vi "Data_Collection.vi"() -> ()   [LabVIEW 2016]
uses:
  <vilib>/Analysis/3filter.llb/Filter Passband Type.ctl
  <vilib>/myRIO/Instrument Drivers/Onboard Devices/Accelerometer/typedefs/Accelerometer Reference.ctl
  <vilib>/myRIO/Common/Instrument Driver Framework/Utilities/typedefs/myRIO Generic Hardware Reference.ctl
  <vilib>/myRIO/Common/Instrument Driver Framework/Utilities/typedefs/Hardware Version Enum.ctl
  <vilib>/myRIO/Common/Instrument Driver Framework/Utilities/typedefs/myRIO v1.0 Reference.ctl
  <vilib>/myRIO/Common/Instrument Driver Framework/Utilities/typedefs/Generic FPGA Reference.ctl
  <vilib>/myRIO/Common/Instrument Driver Framework/myRIO v1.0/Accelerometer/typedefs/Accelerometer Channels List.ctl
  <vilib>/myRIO/Common/Instrument Driver Framework/myRIO v1.0/Accelerometer/typedefs/Accelerometer Channels Enum.ctl
  <vilib>/userdefined/High Color/nirio_resource_hc.ctl
  <vilib>/myRIO/Common/Instrument Driver Framework/Utilities/vis/Is FPGA Ref Available.vi
  <vilib>/myRIO/Common/Instrument Driver Framework/myRIO v1.0/Accelerometer/vis/myRIO v1.1 Open Accelerometer.vi
  <vilib>/myRIO/Instrument Drivers/Onboard Devices/Accelerometer/vis/Read.vi
  <vilib>/myRIO/Common/Instrument Driver Framework/Utilities/vis/Validate Channels.vi
  <vilib>/myRIO/Common/Instrument Driver Framework/myRIO v1.0/Accelerometer/vis/myRIO v1.0 Reserve Accelerometer.vi
  <vilib>/myRIO/Common/Instrument Driver Framework/myRIO v1.0/UART/vis/myRIO v1.0 Close UART.vi
  <vilib>/myRIO/Common/Instrument Driver Framework/myRIO v1.0/Resource Manager/vis/myRIO v1.0 Reserve Channel List.vi
  <vilib>/myRIO/Common/Instrument Driver Framework/myRIO v1.0/Accelerometer/vis/myRIO v1.0 Build MUX Configuration Accelerometer.vi
  <vilib>/myRIO/Common/Instrument Driver Framework/myRIO v1.0/Resource Manager/vis/myRIO v1.0 Reserve Channel.vi
  <vilib>/myRIO/Common/Instrument Driver Framework/myRIO v1.0/Resource Manager/vis/myRIO v1.0 Unreserve Channel.vi
  <vilib>/myRIO/Common/Instrument Driver Framework/myRIO v1.0/Resource Manager/vis/myRIO v1.0 Build Mutex Name.vi
  <vilib>/Utility/VariantDataType/GetNumericInfo.vi
  <vilib>/Utility/error.llb/Error Cluster From Error Code.vi
  <vilib>/myRIO/Common/Instrument Driver Framework/myRIO v1.0/myRIO v1.1 Open.vi
  <vilib>/myRIO/Common/Instrument Driver Framework/myRIO v1.0/Accelerometer/vis/myRIO v1.0 Get Scaling Constant Accelerometer.vi
  <vilib>/myRIO/Common/Instrument Driver Framework/Utilities/vis/IO Manager.vi
  <vilib>/myRIO/Common/Instrument Driver Framework/Utilities/vis/Configuration Manager.vi
  <vilib>/myRIO/Common/Instrument Driver Framework/myRIO v1.0/myRIO v1.0 Close.vi
  <vilib>/myRIO/Common/Instrument Driver Framework/myRIO v1.0/Accelerometer/vis/myRIO v1.0 Read Accelerometer.vi
  <vilib>/myRIO/Common/Instrument Driver Framework/Utilities/vis/FPGA Ref Manager.vi
  <vilib>/myRIO/Common/Instrument Driver Framework/myRIO v1.0/myRIO v1.0 Reset FPGA.vi
  <vilib>/myRIO/Common/Instrument Driver Framework/myRIO v1.0/IRQ/vis/myRIO v1.0 IRQ Info FGV.vi
  <vilib>/myRIO/Common/Instrument Driver Framework/myRIO v1.0/IRQ/vis/myRIO v1.0 Timer IRQ Info FGV.vi
  <vilib>/myRIO/Common/Instrument Driver Framework/myRIO v1.0/IRQ/vis/myRIO v1.0 ISR Agent.vi
  <vilib>/myRIO/Express VI/Onboard Devices/Accelerometer/Accelerometer Express VI.xnode
  <vilib>/myRIO/Instrument Drivers/Onboard Devices/Accelerometer/vis/myRIO Accelerometer Open.xnode
  <vilib>/Analysis/NI_AALBase.lvlib
  <vilib>/myRIO/Instrument Drivers/Onboard Devices/Accelerometer/Accelerometer.lvlib
  <vilib>/ptbypt/NI_PtbyPt.lvlib
  <vilib>/myRIO/Instrument Drivers/Utilities/Utilities.lvlib
panel:
  out "Collected output":dbl[](array[numeric])
  in  "N Samples":dbl
  out "Collected Data":dbl[][](array[numeric])
  in  "Stop Main":bool
  in  "Input Number":dbl
  out "Data as 1D":dbl[](array[numeric])
  out "Data as 2D":dbl[][](array[numeric])
  in  "Start Data Collect":bool
  out "error out":errorcluster
  out "Raw Values":T1(graph) caption="Waveform Chart"
  in  "Stop Data Collect":bool
  out "Pitch and Roll":cluster{"r":dbl, "p":dbl}(graph) caption="Waveform Chart"
  out "?":dbl
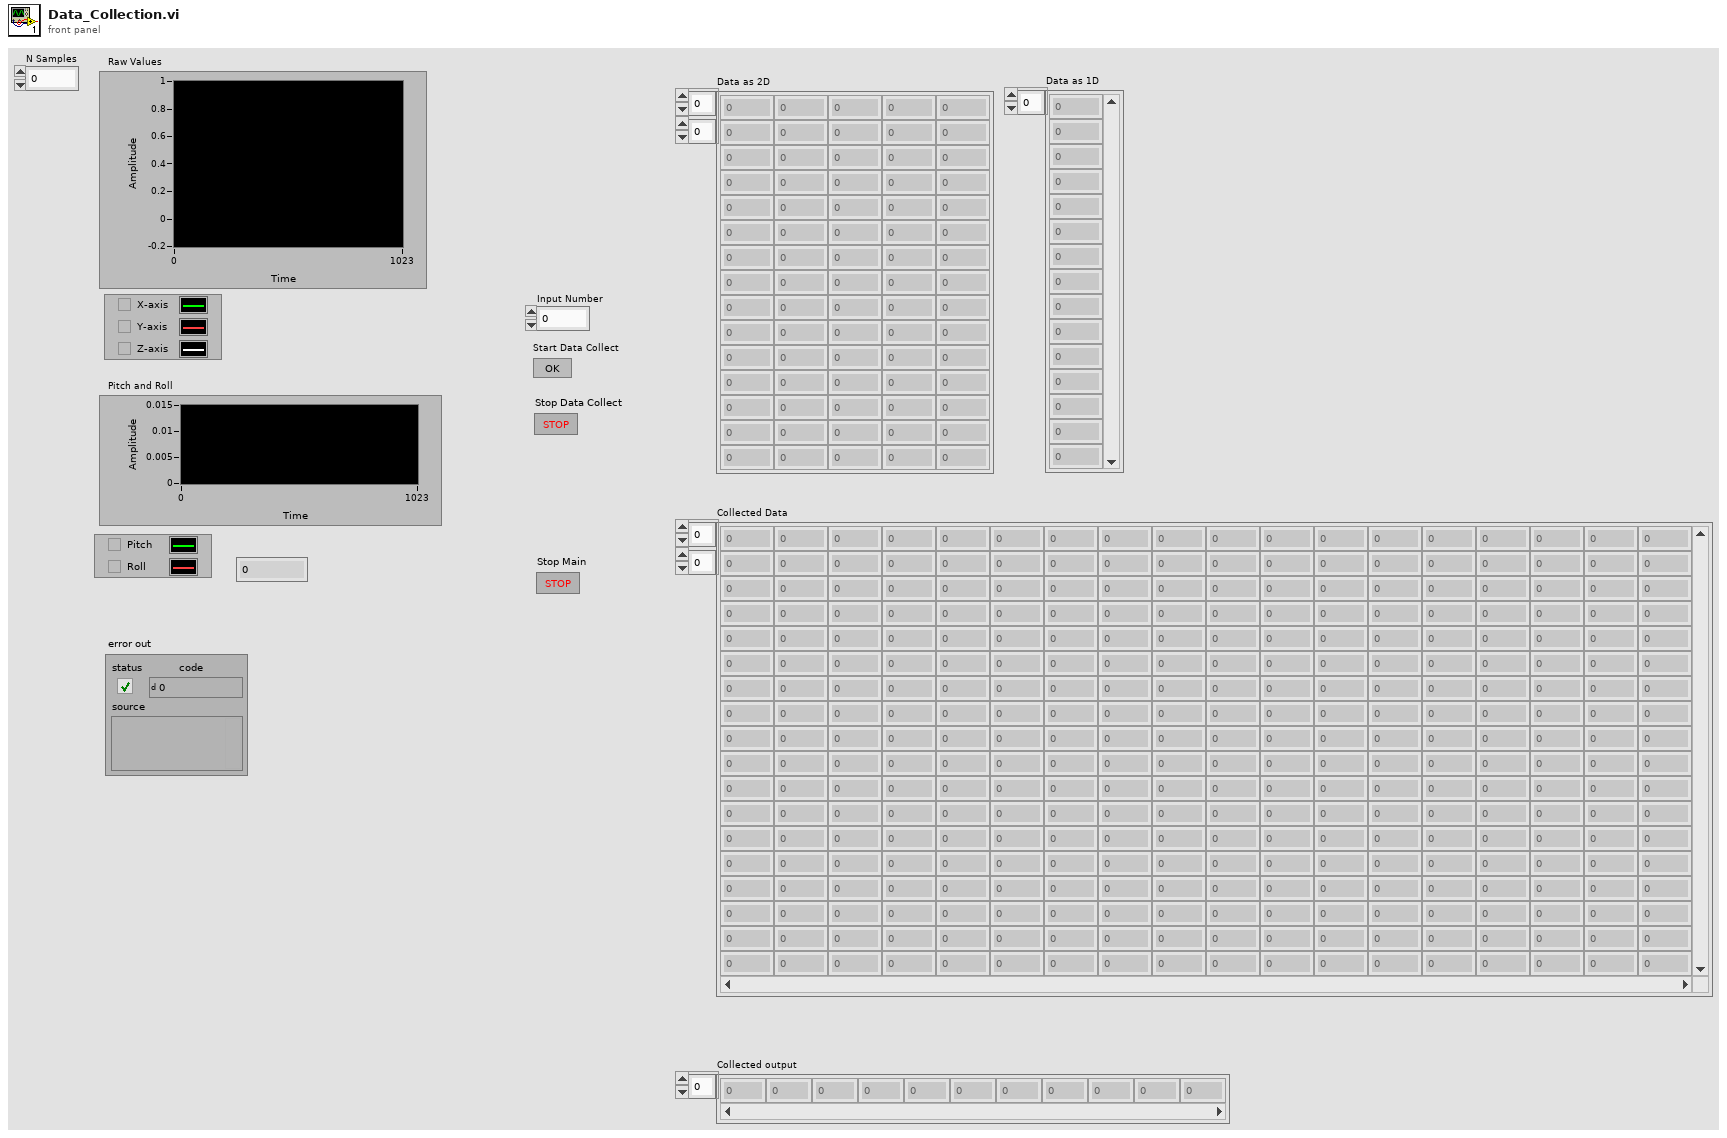
[diagram p1: front panel]
types:
  T1 = cluster{"X-Axis":dbl, "Y-Axis":dbl, "Z-Axis":dbl}
  T2 = typedef "Accelerometer.lvlib/Accelerometer Reference.ctl" = cluster{"myRIO Reference":T3, "Accelerometer Channels List":T7, "LSB Weight":dbl}
  T3 = typedef "myRIO Generic Hardware Reference.ctl" = cluster{"myRIO Model":T4, "myRIO Hardware Reference":T5}
  T4 = typedef "Hardware Version Enum.ctl" = enum16{"Unknown", "myRIO-1900", "myRIO-1950", "roboRIO", "NI ELVIS RIO CM"}
  T5 = typedef "myRIO v1.0 Reference.ctl" = cluster{"Generic FPGA Reference":T6, "Allow multiple opens":bool}
  T6 = typedef "Generic FPGA Reference.ctl" = refnum<k20>
  T7 = typedef "Accelerometer Channels List.ctl" = T8[]
  T8 = typedef "Accelerometer Channels Enum.ctl" = enum16{"Not Connected", "X-Axis", "Y-Axis", "Z-Axis"}
  T9 = typedef "nirio_resource_hc.ctl" = tag
  T10 = typedef "NI_AALBase.lvlib/Filter Passband Type.ctl" = enum32{"Lowpass", "Highpass", "Bandpass", "Bandstop"}
  T11 = cluster{"Filtered x":dbl, "Filtered x":dbl, "Filtered x":dbl}
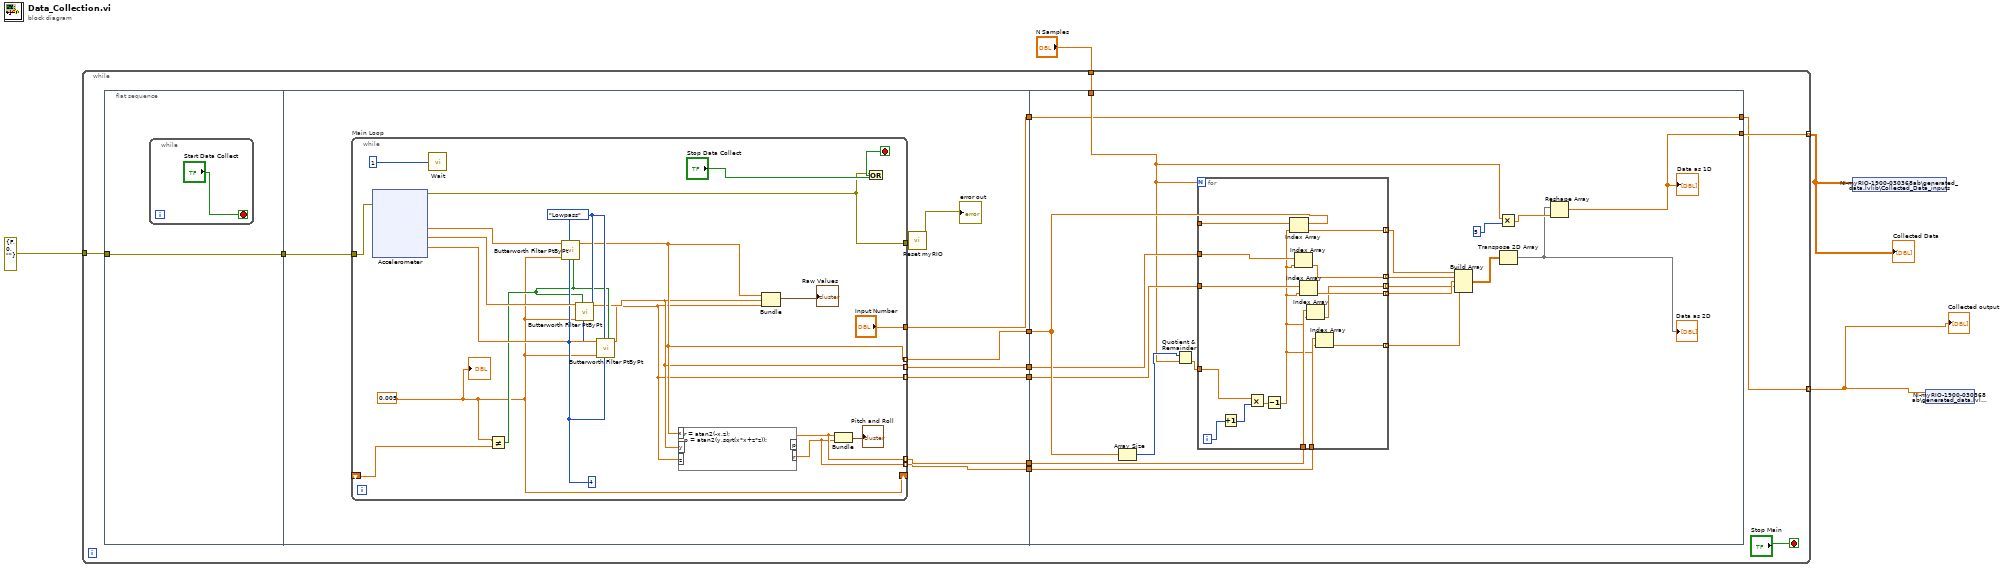
[diagram p0: block diagram]
diagram:
  n1 = while {
    tunnel: errorcluster {"status"=FALSE, "code"=0, "source"=""} ("error in (no error)") -> [w10]
    tunnel: [w8] -> w2 mode=indexing
    tunnel: "N Samples" -> [w7]
    tunnel: [w5] -> w1 mode=indexing
    stop <- "Stop Main" stop-if-true
    n2 = flat-sequence {
      tunnel: w10 -> [w17]
      tunnel: [w17] -> w16
      tunnel: [w25] -> w15
      tunnel: w16 -> [w24]
      tunnel: [w23] -> w14
      tunnel: [w22] -> w13
      tunnel: [w21] -> w12
      tunnel: [w20] -> w11
      tunnel: [w19] -> w6
      tunnel: w15 -> [w105]
      tunnel: w14 -> [w103]
      tunnel: w13 -> [w102]
      tunnel: w12 -> [w101]
      tunnel: w11 -> [w100]
      tunnel: [w90] -> w8
      tunnel: w7 -> [w89]
      tunnel: w6 -> [w88]
      tunnel: [w88] -> w5
      frame #0 {
        n3 = while {
          stop <- "Start Data Collect" stop-if-true
        }
      }
      frame #1 {
        n4 = while "Main Loop" {
          tunnel: [w44] -> w27
          tunnel: w24 -> [w45]
          tunnel: [w41] -> w21 mode=indexing
          tunnel: [w40] -> w20 mode=indexing
          tunnel: [w32] -> w25 mode=indexing
          tunnel: [w31] -> w23 mode=indexing
          tunnel: [w30] -> w22 mode=indexing
          shift-right: [w29] -> _
          shift-left: _ -> [w35]
          tunnel: ["Input Number"] -> w19
          stop <- w46 stop-if-true
          w29 = 0.005
          w36 = 4
          w39 = Filter_Passband_Type."Lowpass" ("filter type")
          n5 = xnode "Accelerometer"("error in (no error)"=w45) -> ("X-Axis"=w33:dbl, "Y-Axis"=w38:dbl, "Z-Axis"=w37:dbl, "error out"=w44:errorcluster)
          n6 = call "Wait"("Count(mSec)"=1) -> ()  [unwired: 1 out]
          n7 = Not Equal?(x=w29, y=w35) -> (x != y?=w34:bool)
          n8 = call <vilib>:"Butterworth Filter PtByPt.vi"("initialize"=w34, "order"=w36, "filter type"=w39, "low cutoff freq: fl"=w29, "x"=w33) -> ("Filtered x"=w32:dbl)  [unwired: 4 in, 1 out]
          n9 = call <vilib>:"Butterworth Filter PtByPt.vi"("initialize"=w34, "order"=w36, "filter type"=w39, "low cutoff freq: fl"=w29, "x"=w38) -> ("Filtered x"=w31:dbl)  [unwired: 4 in, 1 out]
          n10 = call <vilib>:"Butterworth Filter PtByPt.vi"("initialize"=w34, "order"=w36, "filter type"=w39, "low cutoff freq: fl"=w29, "x"=w37) -> ("Filtered x"=w30:dbl)  [unwired: 4 in, 1 out]
          n11 = formula code="r = atan2(-x,z);\np = atan2(y,sqrt(x*x+z*z));"("y"=w31, "z"=w30, "x"=w32) -> ("p"=w41:dbl, "r"=w40:dbl)
          n12 = Bundle("Filtered x"=w32, "Filtered x"=w31, "Filtered x"=w30) -> (→"Raw Values":T11)  [unwired: 1 in]
          n13 = Bundle("p"=w41, "r"=w40) -> (→"Pitch and Roll":cluster{"p":dbl, "r":dbl})  [unwired: 1 in]
          n14 = Or(x=w44, y="Stop Data Collect") -> (x .or. y?=w46:bool)
          "?" <- w29
        }
        n15 = call <vilib>:"Reset myRIO.vi"("error in (no error)"=w27) -> ("error out"=→"error out":errorcluster)  [unwired: 10 in]
      }
      frame #2 {
        n16 = Array Size(array=w105) -> (size(s)=w106:i32)
        n17 = Quotient & Remainder(x=w106, y=w89) -> (floor(x/y)=w104:dbl)  [unwired: 1 out]
        n18 = for {
          N: w89 -> [_]
          tunnel: w105 -> [w118]
          tunnel: w104 -> [w119]
          tunnel: [w117] -> w99 mode=indexing
          tunnel: w103 -> [w116]
          tunnel: w102 -> [w115]
          tunnel: w101 -> [w114]
          tunnel: w100 -> [w113]
          tunnel: [w112] -> w98 mode=indexing
          tunnel: [w111] -> w97 mode=indexing
          tunnel: [w110] -> w96 mode=indexing
          tunnel: [w109] -> w95 mode=indexing
          i -> [w120]
          n19 = Increment(x=w120) -> (x+1=w121:i32)
          n20 = Multiply(x=w119, y=w121) -> (x*y=w108:dbl)
          n21 = Decrement(x=w108) -> (x-1=w107:dbl)
          n22 = Index Array(array=w118, index=w107) -> (element=w117:dbl)
          n23 = Index Array(array=w116, index=w107) -> (element=w112:dbl)
          n24 = Index Array(array=w115, index=w107) -> (element=w111:dbl)
          n25 = Index Array(array=w114, index=w107) -> (element=w110:dbl)
          n26 = Index Array(array=w113, index=w107) -> (element=w109:dbl)
        }
        n27 = Build Array(w99, w98, w97, w96, w95) -> (w94:dbl[][])
        n28 = Multiply(x=w89, y=5) -> (x*y=w92:dbl)
        n29 = Transpose 2D Array(2D array=w94) -> (transposed array=w91:dbl[][])
        "Data as 2D" <- w91
        n30 = Reshape Array(w91, w92) -> (w90:dbl[])
        "Data as 1D" <- w90
      }
    }
  }
  "Collected Data" <- w2
  "Collected output" <- w1
  n31 = shared-variable "NI-myRIO-1900-030368ab\\generated_data.lvlib\\Collected_Data_inputs"(w2) -> ()  [unwired: 1 in, 1 out]
  n32 = shared-variable "NI-myRIO-1900-030368ab\\generated_data.lvlib\\Targets"(w1) -> ()  [unwired: 1 in, 1 out]
